vi "VisionPoseConversions.vi"(6 "Previous Y Estimate (in)":dbl, 7 "Previous X Estimate (in)":dbl, 8 "turret heading [0, 360]":dbl, 9 "robot heading [0,360]":dbl, 10 "LimeLight Raw X (in)":dbl, 11 "LimeLight Raw Z (in)":dbl) -> (2 "deltaY (in)":dbl, 3 "deltaX (in)":dbl)   [LabVIEW 2019]
panel:
  in  "X Offset (in)":dbl=629.25
  in  "Y Offset (in)":dbl=94.66
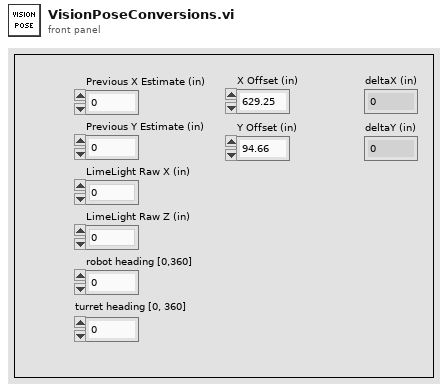
[diagram p1: front panel]
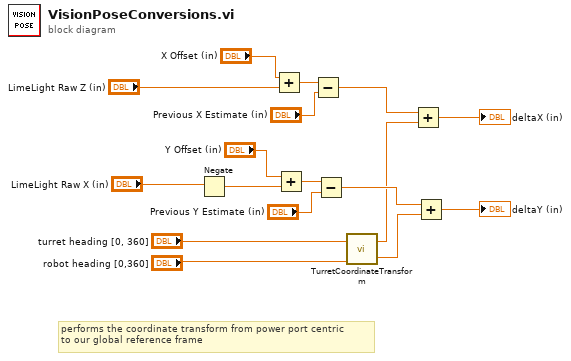
[diagram p0: block diagram]
diagram:
  # "performs the coordinate transform from power port centric\nto our global reference frame"
  n1 = Negate(x="LimeLight Raw X (in)") -> (-x=w17:dbl)
  n2 = Add(x="X Offset (in)", y="LimeLight Raw Z (in)") -> (x+y=w12:dbl)
  n3 = Add(x="Y Offset (in)", y=w17) -> (x+y=w14:dbl)
  n4 = Subtract(x=w12, y="Previous X Estimate (in)") -> (x-y=w2:dbl)
  n5 = Subtract(x=w14, y="Previous Y Estimate (in)") -> (x-y=w5:dbl)
  n6 = call "TurretCoordinateTransform.vi"("robot heading [0,360]"="robot heading [0,360]", "turret heading [0, 360]"="turret heading [0, 360]") -> ("Ly"=w6:dbl, "Lx"=w3:dbl)
  n7 = Add(x=w2, y=w3) -> (x+y=→"deltaX (in)":dbl)
  n8 = Add(x=w5, y=w6) -> (x+y=→"deltaY (in)":dbl)
